vi "Piezo Calibration Param Get.vi"   [LabVIEW 2019, in "Nanonis Prog Interface.lvlib"]
doc: "<B>Returns the piezo range (m) or sensitivity (m/V) values for all 3 axes (X, Y, Z). </B>\n\nThis is a polymorphic funtion where you can select between sensitivity and range of the scan piezo. \n\n- Nanonis Programming Interface -"
uses:
  <userlib>/Nanonis Prog Interface V5/Nanonis Prog Interface.lvlib
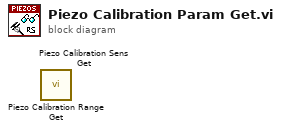
[diagram p0: block diagram]
diagram:
  n1 = call <userlib>:"Piezo Calibration Range Get.vi"() -> ()  [unwired: 11 in, 5 out]
  n2 = call <userlib>:"Piezo Calibration Sens Get.vi"() -> ()  [unwired: 11 in, 5 out]
